vi "system.TestLauncher.vi"() -> ()   [LabVIEW 2016, in "system.lvclass"]
uses:
  system.lvclass
  <vilib>/JKI/JKI SMO/SMO/Typedefs/SMOState --Enum.ctl
  Generator/Typedefs/configGenerator-array-cluster.ctl
  DSP/Typedefs/PrivateEvents--DSP.RunCalculation.ctl
  DSP/Typedefs/LP_Config.ctl
  DSP.lockin/Typedefs/Lockin_Config.ctl
  DSP/Typedefs/FFT_Config.ctl
  <vilib>/Analysis/4window.llb/windowTd.ctl
  <vilib>/measure/maspectr.llb/Power Spectrum and PSD Export Mode.ctl
  <vilib>/JKI/JKI SMO/SMO/SMO.lvclass
  C:/Program Files (x86)/National Instruments/LabVIEW 2016/vi.lib/JKI/JKI SMO/SMO/SMO.lvclass
  Generator/Generator.lvclass
  DSP/DSP.lvclass
  DSP.lockin/DSP_lockin.lvclass
  <vilib>/Analysis/NI_AALPro.lvlib
  <vilib>/measure/NI_MAPro.lvlib
panel:
  in  "runCalculation":T1={"runCalculation"={"adjust gain"=FALSE, "subtract offset"=FALSE, "60 Hz prefilter"=FALSE, "LP prefilter"=FALSE, "lockin"=FALSE, "FFT"=FALSE, "gain"=[], "offset"=[], "LP config"={"high cutoff freq [Hz]"=0.45}, "Lockin config"=[], "FFT config"={"averaging parameters"={"averaging mode"=enum."RMS averaging", "weighting mode"=enum."Exponential", "number of averages"=10}, "window"=1, "export mode"=0, "window parameter"=nan, "restart averaging (F)"=FALSE}}} {"runCalculation"."FFT config"."export mode" items=["Power Spectrum", "Power Spectral Density"]; "runCalculation"."FFT config"."window" items=["Rectangle"=0, "Hanning"=1, "Hamming"=2, "Blackman-Harris"=3, "Exact Blackman"=4, "Blackman"=5, "Flat Top"=6, "4 Term B-Harris "=7, "7 Term B-Harris"=8, "Low Sidelobe"=9, "Blackman Nuttall"=11, "Triangle"=30, "Bartlett-Hanning"=31, "Bohman"=32, "Parzen"=33, "Welch"=34, "Kaiser"=60, "Dolph-Chebyshev"=61, "Gaussian"=62]; "runCalculation"."FFT config"."averaging parameters"."number of averages" min=1; "runCalculation"."Lockin config"."TC (s)" format="%#_13g"}
  in  "Channel":dbl
  out "Y/R":dbl format="%#_6p"
  out "X/R":dbl format="%#_6p"
  out "Waveform Chart 2":waveform(dbl)[](graph)
  out "Waveform Chart":waveform(dbl)[](graph)
  in  "Display":enum16{"X and Y", "R and Theta"}(ring)=enum."R and Theta"
  out "REF":waveform(dbl)[](graph)
  in  "output config":T7
  out "Write":T8(graph)
  out "Read":waveform(dbl)[](graph)
  out "SMO State":T9
  out "error out":errorcluster
  in  "Stop":bool
  # "LOCKIN: Basic SMO Test Launcher: OBSOLETE!!!! REPLACE WITH APPLAUNCHER"
  # "LOCKIN: Basic SMO Test Launcher"
  # "For instructions on how to use the JKI State Machine Objects, examples and video tutorials, visit:\nhttp://jki.net/state-machine-objects/\n\nJKI State Machine Objects™\nhttp://jki.net/state-machine-objects/\nCopyright (C) 2005-2015, JKI <info@jki.net>\nALL RIGHTS RESERVED"
  # "should make call directly to lockin"
  # "use network streams to pass data between different computers?\nOr ZeroMQ?\nhave lockin running on different (or same) computers\none is AO/AI\nThe other is lockin DSP"
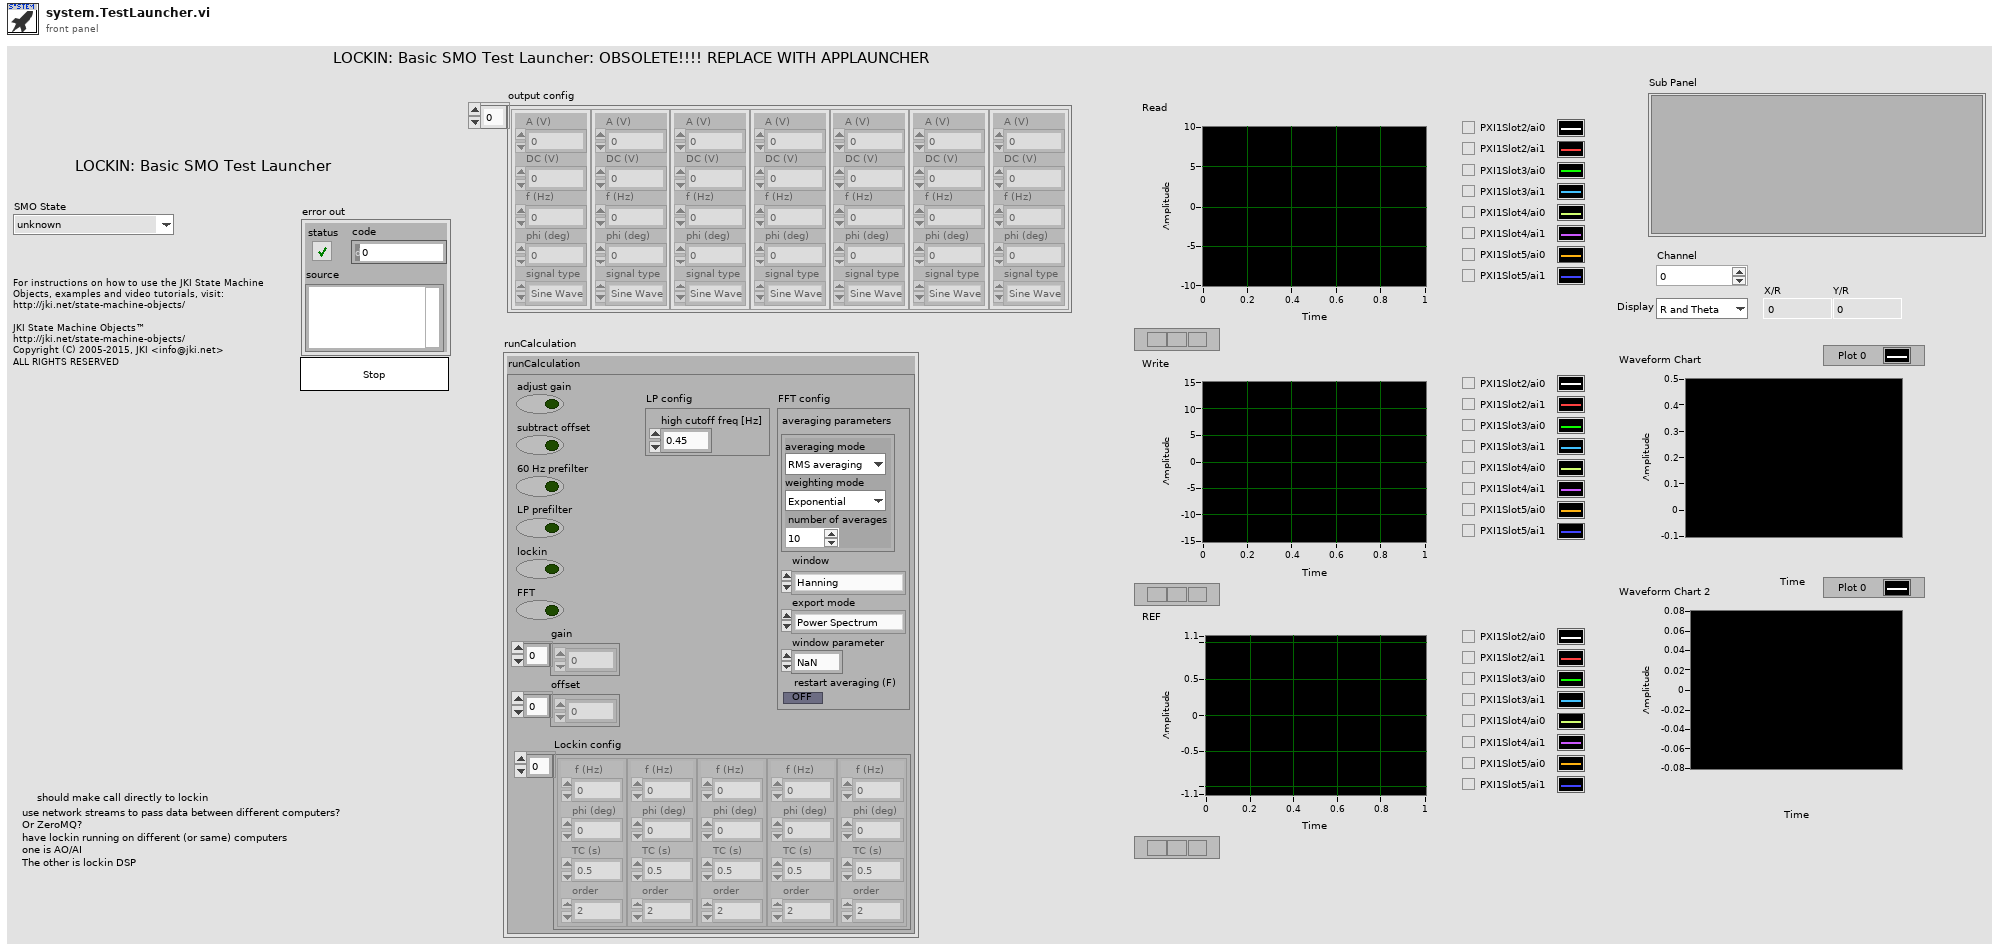
[diagram p1: front panel]
types:
  T1 = typedef "DSP.lvclass/PrivateEvents--DSP.RunCalculation.ctl" = cluster{"runCalculation":cluster{"adjust gain":bool, "subtract offset":bool, "60 Hz prefilter":bool, "LP prefilter":bool, "lockin":bool, "FFT":bool, "gain":dbl[], "offset":dbl[], "LP config":T2, "Lockin config":T3, "FFT config":T4}}
  T2 = typedef "DSP.lvclass/LP_Config.ctl" = cluster{"high cutoff freq [Hz]":dbl}
  T3 = typedef "DSP_lockin.lvclass/Lockin_Config.ctl" = cluster{" f (Hz)":dbl, "phi (deg)":dbl, "TC (s)":dbl, "order":i32}[]
  T4 = typedef "DSP.lvclass/FFT_Config.ctl" = cluster{"averaging parameters":cluster{"averaging mode":enum16{"No averaging", "Vector averaging", "RMS averaging", "Peak hold"}, "weighting mode":enum16{"Linear", "Exponential"}, "number of averages":u32}, "window":T5, "export mode":T6, "window parameter":dbl, "restart averaging (F)":bool}
  T5 = typedef "NI_AALPro.lvlib/windowTd.ctl" = u32
  T6 = typedef "NI_MAPro.lvlib/Power Spectrum and PSD Export Mode.ctl" = u16
  T7 = typedef "Generator.lvclass/configGenerator-array-cluster.ctl" = cluster{"A (V)":dbl, "DC (V)":dbl, "f (Hz)":dbl, "phi (deg)":dbl, "signal type":enum16{"Sine Wave", "Triangle Wave", "Square Wave", "Sawtooth Wave"}}[]
  T8 = typedef "system.lvclass/PublicEvents--lockin.Write.ctl" = waveform(dbl)[]
  T9 = typedef "SMO.lvclass/SMOState --Enum.ctl" = enum16{"unknown", "Created", "Started", "Stopped"}
  T10 = typedef "SMO.lvclass/Public Events.ctl" = cluster{"Error":refnum<user-event>, "State":refnum<user-event>, "Reserve State":refnum<user-event>}
  T11 = typedef "system.lvclass/PublicEvents--Cluster.ctl" = cluster{"read":refnum<user-event>, "Write":refnum<user-event>, "lockin_REF_waveform":refnum<user-event>, "lockin_results":refnum<user-event>}
  T12 = cluster{"Event Registration Refnum":refnum<event-registration>}
  T13 = typedef "system.lvclass/PublicEvents--lockin.read.ctl" = waveform(dbl)[]
  T14 = typedef "system.lvclass/PublicEvents--lockin.lockin_REF_waveform.ctl" = waveform(dbl)[]
  T15 = typedef "system.lvclass/PublicEvents--lockin.lockin_results.ctl" = dbl[][]
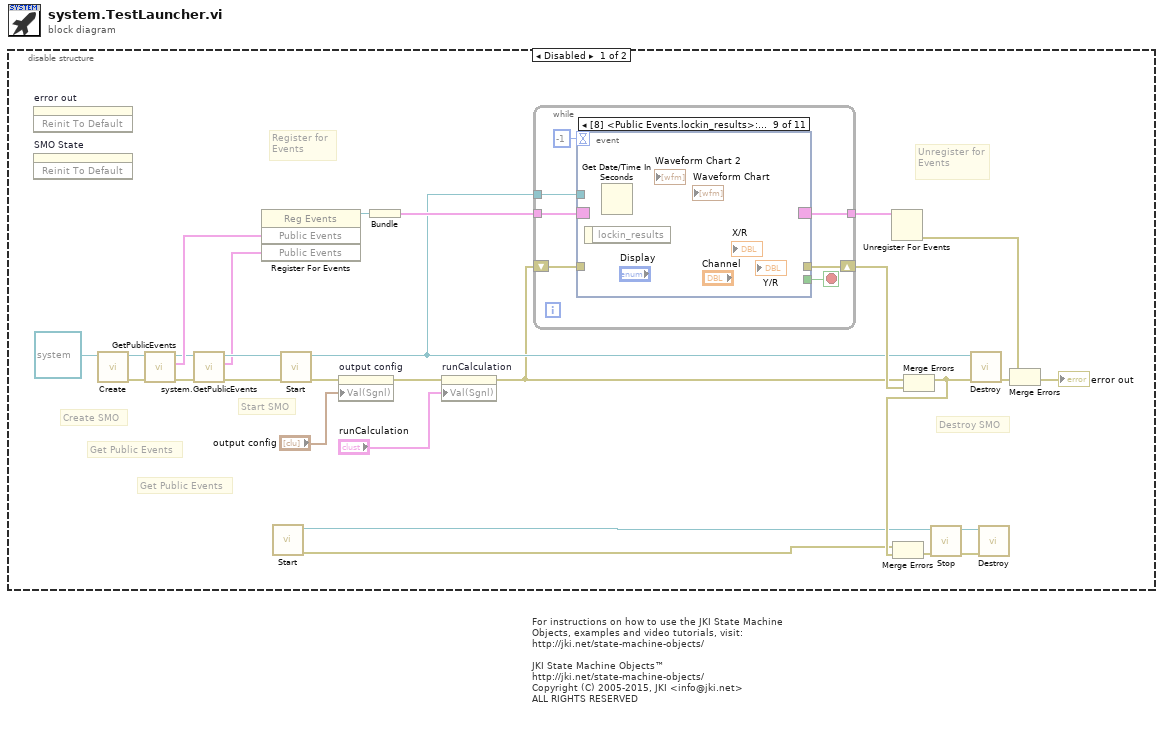
[diagram p0: block diagram]
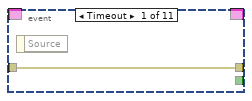
[diagram p2: hidden frame]
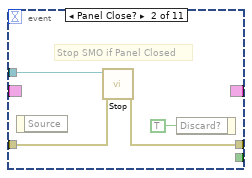
[diagram p3: hidden frame]
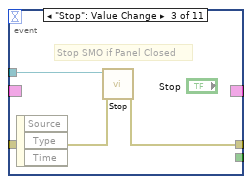
[diagram p4: hidden frame]
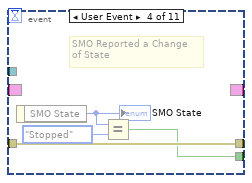
[diagram p5: hidden frame]
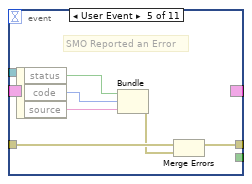
[diagram p6: hidden frame]
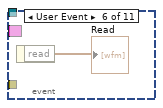
[diagram p7: hidden frame]
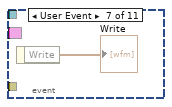
[diagram p8: hidden frame]
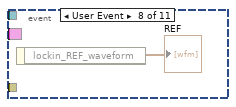
[diagram p9: hidden frame]
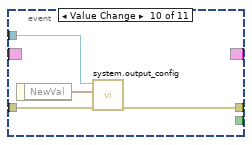
[diagram p10: hidden frame]
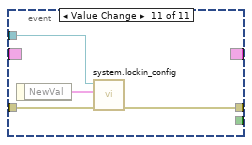
[diagram p11: hidden frame]
diagram:
  # "For instructions on how to use the JKI State Machine Objects, examples and video tutorials, visit:\nhttp://jki.net/state-machine-objects/\n\nJKI State Machine Objects™\nhttp://jki.net/state-machine-objects/\nCopyright (C) 2005-2015, JKI <info@jki.net>\nALL RIGHTS RESERVED"
  n1 = disable-structure shown="Disabled" {
    frame Disabled {
      # "Get Public Events"
      # "Get Public Events"
      # "Start SMO"
      # "Destroy SMO"
      # "Create SMO"
      # "Unregister for Events"
      # "Register for Events"
      n2 = invoke on="error out" class="Clust (strict)" method="Reinit To Default"() -> ()  [unwired: 3 in, 3 out]
      n3 = invoke on="SMO State" class="Enum (strict)" method="Reinit To Default"() -> ()  [unwired: 3 in, 3 out]
      n4 = call <vilib>:"Create.vi"("SMO"=refnum<class "system.lvclass"> refnum ("SMO.Template.lvclass")) -> ("error out"=w21:errorcluster, "SMO out"=w22:refnum<class "system.lvclass">)  [unwired: 8 in, 1 out]
      n5 = call <vilib>:"GetPublicEvents.vi"("error in (no error)"=w21, "SMO"=w22) -> ("error out"=w17:errorcluster, "Public Events"=w20:T10, "SMO out"=w18:refnum<class "system.lvclass">)  [unwired: 7 in]
      n6 = call "system.GetPublicEvents.vi"("error in (no error)"=w17, "lockin"=w18) -> ("error out"=w15:errorcluster, "Public Events"=w11:T11, "lockin out"=w16:refnum<class "system.lvclass">)  [unwired: 7 in]
      n7 = register-events(w20, w11) -> (reference out=w19:refnum<event-registration>)  [unwired: 2 in, 1 out]
      n8 = call <vilib>:"Start.vi"() -> ("error out"=w3:errorcluster, "SMO out"=w2:refnum<class "SMO.lvclass">)  [unwired: 10 in]
      n9 = call <vilib>:"Start.vi"("error in (no error)"=w15, "SMO"=w16) -> ("error out"=w13:errorcluster, "SMO out"=w14:refnum<class "system.lvclass">)  [unwired: 8 in]
      n10 = property on="output config" class="Arr (strict)"(error in=w13, "Val(Sgnl)"="output config") -> (error out=w10:errorcluster)  [unwired: 1 in, 1 out]
      n11 = Bundle("Event Registration Refnum"=w19) -> (w27:T12)  [unwired: 1 in]
      n12 = property on="runCalculation" class="Clust (strict)"(error in=w10, "Val(Sgnl)"="runCalculation") -> (error out=w9:errorcluster)  [unwired: 1 in, 1 out]
      n13 = while {
        shift-right: [w34] -> w26
        shift-left: w9 -> [w33]
        tunnel: w27 -> [w32]
        tunnel: [w31] -> w28
        tunnel: w14 -> [w30]
        stop <- w35 stop-if-true
        n14 = event shown="[8] <Public Events.lockin_results>: User Event" {
          selector: w32 -> [_ _ _ _ _ _ _ _ _ _ _]
          dyn-events: [_ _ _ _ _ _ _ _ _ _ _] -> w31
          timeout: -1 -> [_ _ _ _ _ _ _ _ _ _ _]
          tunnel: [_ _ _ w44 _ _ _ _ _ _ _] -> w35
          tunnel: w30 -> [_ w40 w43 _ _ _ _ _ _ w64 w70]
          tunnel: [w36 w39 w42 w47 w51 _ _ _ _ w65 w68] -> w34
          tunnel: w33 -> [w36 w38 w41 w47 w49 _ _ _ _ w66 w69]
          event Timeout {
            n15 = event-data() -> ()  [unwired: 1 in, 1 out]
          }
          event Panel Close? {
            # "Stop SMO if Panel Closed"
            n16 = event-data() -> ()  [unwired: 1 in, 1 out]
            n17 = call <vilib>:"Stop.vi"("error in (no error)"=w38, "SMO"=w40) -> ("error out"=w39:errorcluster)  [unwired: 8 in, 1 out]
            n18 = event-data("Discard?"=TRUE ("OK")) -> ()  [unwired: 1 in, 1 out]
          }
          event "Stop": Value Change {
            # "Stop SMO if Panel Closed"
            n19 = event-data() -> ()  [unwired: 1 in, 3 out]
            n20 = call <vilib>:"Stop.vi"("error in (no error)"=w41, "SMO"=w43) -> ("error out"=w42:errorcluster)  [unwired: 8 in, 1 out]
          }
          event User Event {
            # "SMO Reported a Change\nof State"
            n21 = event-data() -> ("SMO State"=w46:T9)  [unwired: 1 in]
            "SMO State" <- w46
            n22 = Equal?(x=w46, y=SMOState_--Enum."Stopped") -> (x = y?=w44:bool)
          }
          event User Event {
            # "SMO Reported an Error"
            n23 = event-data() -> ("status"=w50:bool, "code"=w53:i32, "source"=w52:string)  [unwired: 1 in]
            n24 = Bundle("status"=w50, "code"=w53, "source"=w52) -> (w48:errorcluster)  [unwired: 1 in]
            n25 = Merge Errors(w49, w48) -> (w51:errorcluster)
          }
          event User Event {
            n26 = event-data() -> ("read"=→"Read":T13)  [unwired: 1 in]
          }
          event User Event {
            n27 = event-data() -> ("Write"=→"Write":T8)  [unwired: 1 in]
          }
          event User Event {
            n28 = event-data() -> ("lockin_REF_waveform"=→"REF":T14)  [unwired: 1 in]
          }
          event User Event {
            n29 = event-data() -> ("lockin_results"=w62:T15)  [unwired: 1 in]
            n30 = Get Date/Time In Seconds() -> (seconds since 1Jan1904=w57:timestamp)
          }
          event Value Change {
            n31 = event-data() -> ("NewVal"=w63:T7)  [unwired: 1 in]
            n32 = call "system.output_config.vi"("error in (no error)"=w66, "output_config"=w63, "lockin"=w64) -> ("error out"=w65:errorcluster)  [unwired: 7 in, 1 out]
          }
          event Value Change {
            n33 = event-data() -> ("NewVal"=w67:T1)  [unwired: 1 in]
            n34 = call "system.lockin_config.vi"("error in (no error)"=w69, "runCalculation"=w67, "lockin"=w70) -> ("error out"=w68:errorcluster)  [unwired: 7 in, 1 out]
          }
        }
      }
      n35 = Unregister For Events(event registration refnum=w28) -> (error out=w25:errorcluster)  [unwired: 1 in]
      n36 = Merge Errors(w9, w26) -> (w5:errorcluster)
      n37 = Merge Errors(w3, w5) -> (w4:errorcluster)
      n38 = call <vilib>:"Stop.vi"("error in (no error)"=w4, "SMO"=w2) -> ("error out"=w6:errorcluster, "SMO out"=w7:refnum<class "SMO.lvclass">)  [unwired: 8 in]
      n39 = call <vilib>:"Destroy.vi"("error in (no error)"=w5, "SMO"=w14) -> ("error out"=w23:errorcluster)  [unwired: 9 in]
      n40 = call <vilib>:"Destroy.vi"("error in (no error)"=w6, "SMO"=w7) -> ()  [unwired: 9 in, 1 out]
      n41 = Merge Errors(w25, w23) -> (→"error out":errorcluster)
    }
    frame Enabled {
    }
  }
